vi "TCParseLeidenComputerNames.vi"(8 "error in (no error)":errorcluster, 9 "AVS type":T1(ring) caption="Bridge Type", 10 "computer name":string="custardpie") -> (0 "error out":errorcluster, 1 "AVS Type":T2(ring)=enum."CF_Z_Bridge")   [LabVIEW 2013]
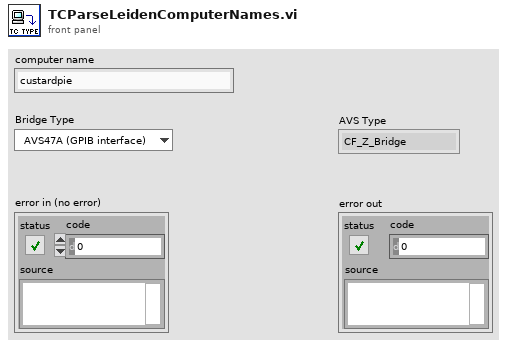
[diagram p1: front panel]
types:
  T1 = enum16{"AVS47A (GPIB interface)", "AVS47B (RS232 interface)", "AVS48", "AVS Emulation", "Impedance Bridge", "Disabled"}
  T2 = enum16{"CF", "CF_Z_Bridge", "MNK", "MNK_Z_Bridge"}
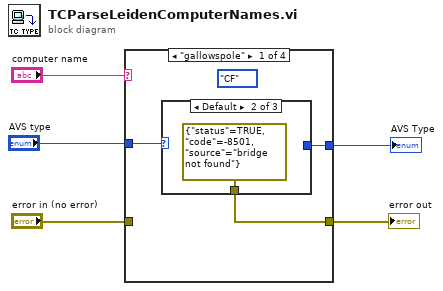
[diagram p0: block diagram]
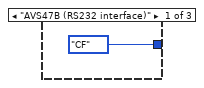
[diagram p2: hidden frame]
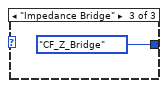
[diagram p3: hidden frame]
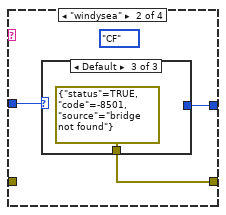
[diagram p4: hidden frame]
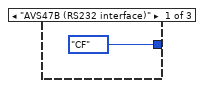
[diagram p5: hidden frame]
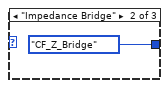
[diagram p6: hidden frame]
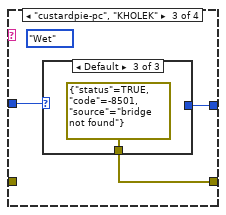
[diagram p7: hidden frame]
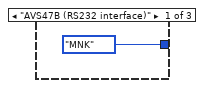
[diagram p8: hidden frame]
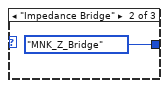
[diagram p9: hidden frame]
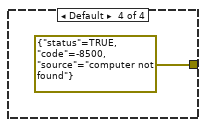
[diagram p10: hidden frame]
diagram:
  n1 = case shown="\"gallowspole\"" "computer name" {
    tunnel: "error in (no error)" -> [_ _ _ _]
    tunnel: [w6 w12 w18 errorcluster {"status"=TRUE, "code"=-8500, "source"="computer not found"} ("error in (no error)")] -> w3
    tunnel: "AVS type" -> [w8 w13 w19 _]
    tunnel: [w7 w14 w20 _] -> w1
    frame "gallowspole" {
      (unwired) enum32{"CF", "Wet"}."CF" ("Type")
      n2 = case shown="Default" w8 {
        tunnel: [T2."CF" ("AVS Type") _ T2."CF_Z_Bridge" ("AVS Type")] -> w7
        tunnel: [_ errorcluster {"status"=TRUE, "code"=-8501, "source"="bridge not found"} ("error in (no error)") _] -> w6
        frame "AVS47B (RS232 interface)" {
        }
        frame Default {
        }
        frame "Impedance Bridge" {
        }
      }
    }
    frame "windysea" {
      (unwired) enum32{"CF", "Wet"}."CF" ("Type")
      n3 = case shown="Default" w13 {
        tunnel: [T2."CF" ("AVS Type") T2."CF_Z_Bridge" ("AVS Type") _] -> w14
        tunnel: [_ _ errorcluster {"status"=TRUE, "code"=-8501, "source"="bridge not found"} ("error in (no error)")] -> w12
        frame "AVS47B (RS232 interface)" {
        }
        frame "Impedance Bridge" {
        }
        frame Default {
        }
      }
    }
    frame "custardpie-pc", "KHOLEK" {
      (unwired) enum32{"CF", "Wet"}."Wet" ("Type")
      n4 = case shown="Default" w19 {
        tunnel: [T2."MNK" ("AVS Type") T2."MNK_Z_Bridge" ("AVS Type") _] -> w20
        tunnel: [_ _ errorcluster {"status"=TRUE, "code"=-8501, "source"="bridge not found"} ("error in (no error)")] -> w18
        frame "AVS47B (RS232 interface)" {
        }
        frame "Impedance Bridge" {
        }
        frame Default {
        }
      }
    }
    frame Default {
    }
  }
  "error out" <- w3
  "AVS Type" <- w1
